vi "GT Get Follow Master.vi"(0 "cardNum":i16, 1 "pMasterItem":i16, 5 "profile":i16, 7 "pMasterIndex":i16, 9 "pMasterType":i16, 11 "error in (no error)":errorcluster caption="错误输入（无错误）") -> (3 "pMasterItem out":i16, 4 "function return":i16, 8 "pMasterIndex out":i16, 10 "pMasterType out":i16, 15 "error out":errorcluster caption="错误输出")   [LabVIEW 2014, in "gts.lvlib"]
doc: "GT_API GT_GetFollowMaster(short cardNum,short profile,short *pMasterIndex,short *pMasterType=NULL,short *pMasterItem=NULL);"
uses:
  gts.lvlib
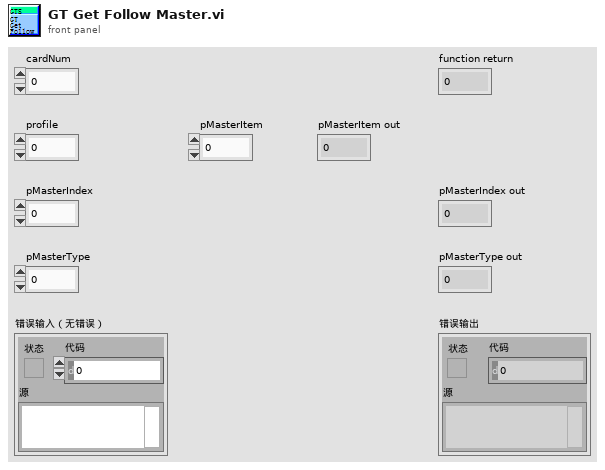
[diagram p1: front panel]
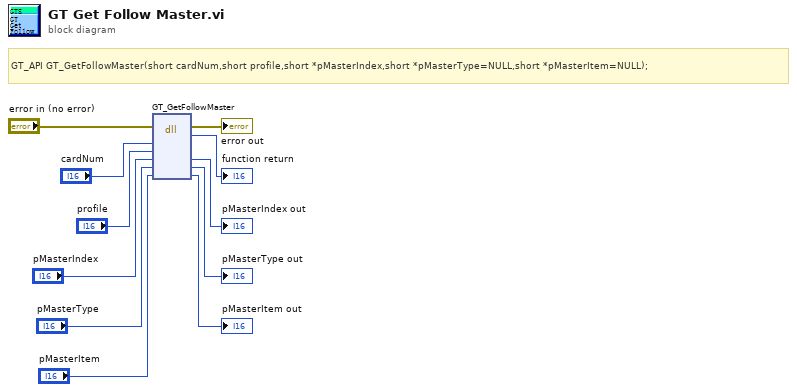
[diagram p0: block diagram]
diagram:
  # "GT_API GT_GetFollowMaster(short cardNum,short profile,short *pMasterIndex,short *pMasterType=NULL,short *pMasterItem=NULL);"
  n1 = dll-call lib="PTH2habs D固高科技资料GTS控制卡GTS卡18年上半年资料dllVC32bit\nmulti_cardgts.*" fn="GT_GetFollowMaster"(error in="error in (no error)", "cardNum"="cardNum", "profile"="profile", "pMasterIndex"="pMasterIndex", "pMasterType"="pMasterType", "pMasterItem"="pMasterItem") -> (error out=→"error out":errorcluster, →"function return":i16, "pMasterIndex"=→"pMasterIndex out":i16, "pMasterType"=→"pMasterType out":i16, "pMasterItem"=→"pMasterItem out":i16)  [unwired: 4 in, 1 out]
